vi "Mean.vi"(8 "error in (no error)":errorcluster, 10 "y":dbl, 11 "x":dbl) -> (0 "error out":errorcluster, 2 "out":dbl)   [LabVIEW 2011]
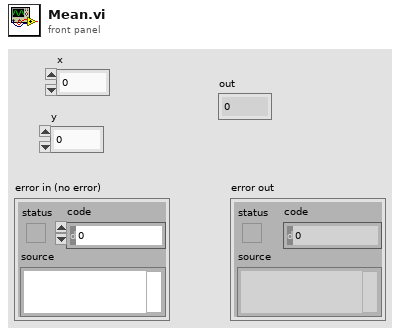
[diagram p1: front panel]
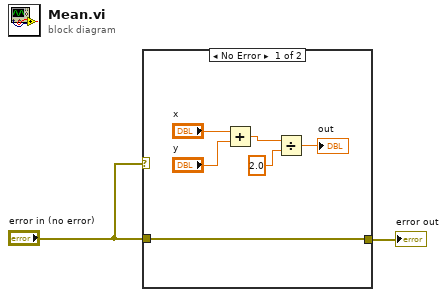
[diagram p0: block diagram]
diagram:
  n1 = case shown="No Error" "error in (no error)" {
    tunnel: [w3 w9] -> w1
    tunnel: "error in (no error)" -> [w3 w9]
    frame No Error {
      n2 = Add(x="x", y="y") -> (x+y=w6:dbl)
      n3 = Divide(x=w6, y=2.0) -> (x/y=→"out":dbl)
    }
    frame Error {
    }
  }
  "error out" <- w1
